vi "Write Folder Path.vi"(8 "error in (no error)":errorcluster, 10 "Folder Path":path, 11 "Tree Data Folder in":refnum<class "Tree Data Folder.lvclass">) -> (0 "error out":errorcluster, 3 "Tree Data Folder out":refnum<class "Tree Data Folder.lvclass">)   [LabVIEW 2024, in "Tree Data Folder.lvclass"]
uses:
  Tree Data Folder.lvclass
  Tree Data Folder.lvclass/Tree Data Folder.ctl
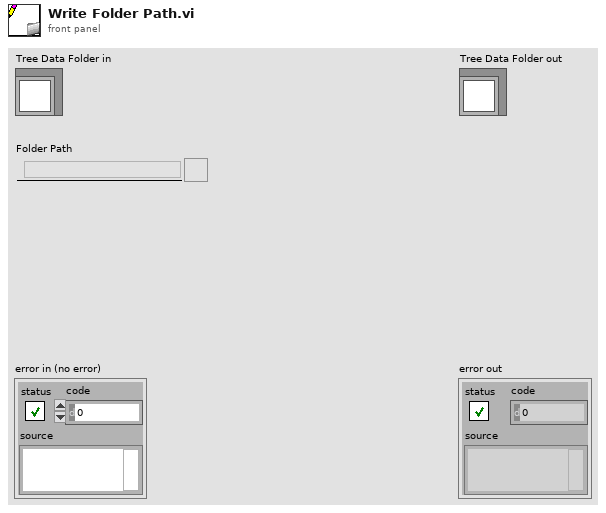
[diagram p1: front panel]
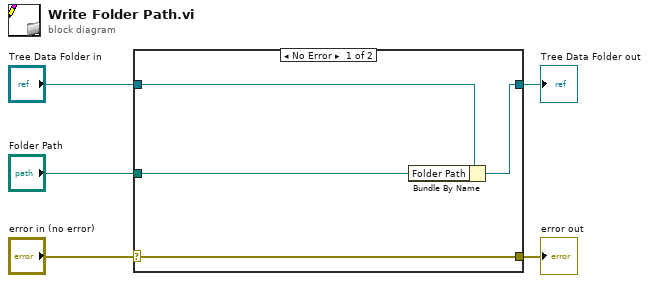
[diagram p0: block diagram]
diagram:
  n1 = case shown="No Error" "error in (no error)" {
    selector: "error in (no error)" -> [w9 w10]
    tunnel: [w9 w10] -> w4
    tunnel: [w7 w11] -> w2
    tunnel: "Tree Data Folder in" -> [w8 w11]
    tunnel: "Folder Path" -> [w6 _]
    frame No Error {
      n2 = Bundle By Name(cluster=w8, "Folder Path"=w6) -> (w7:refnum<class "Tree Data Folder.lvclass">)
    }
    frame Error {
    }
  }
  "error out" <- w4
  "Tree Data Folder out" <- w2
